vi "Source_Q_wrong.vi"(2 "Ch Names":string[](array[string]), 3 "Values":dbl[](array[numeric]) format="%.2f") -> (0 "Gas Error?":bool)   [LabVIEW 2010]
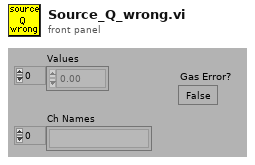
[diagram p1: front panel]
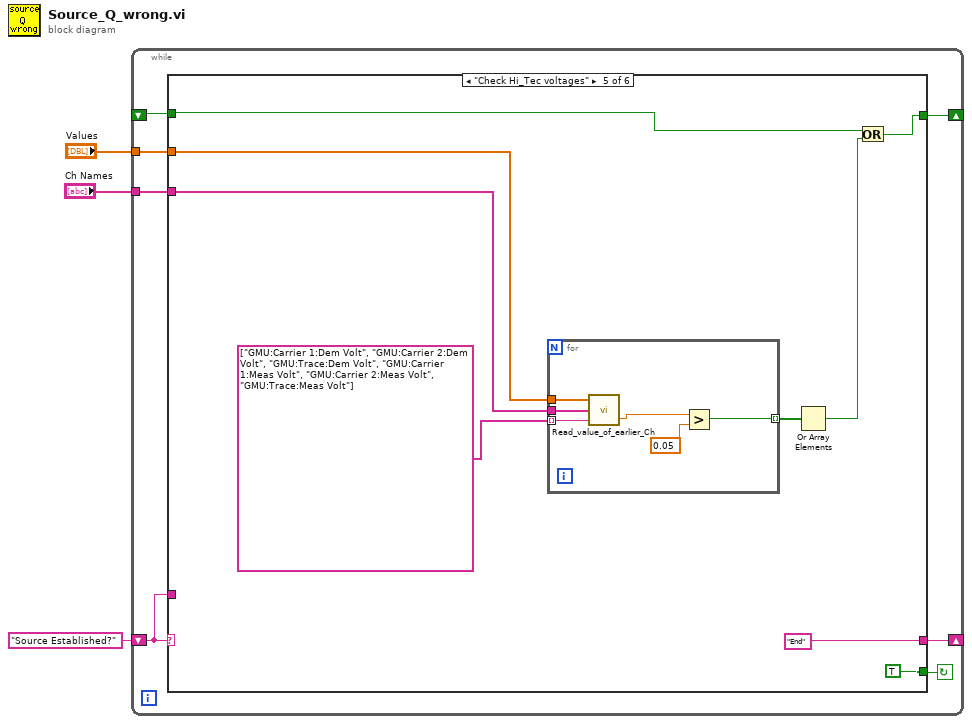
[diagram p0: block diagram]
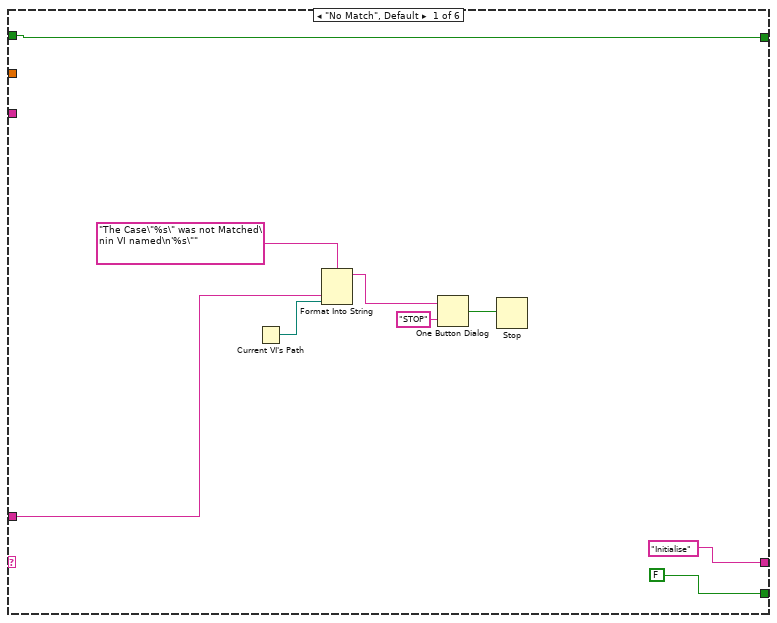
[diagram p2: hidden frame]
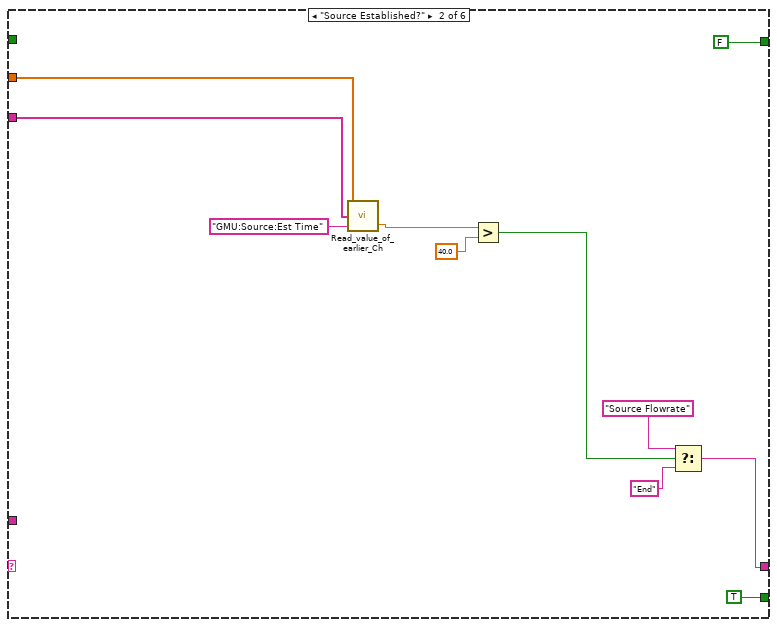
[diagram p3: hidden frame]
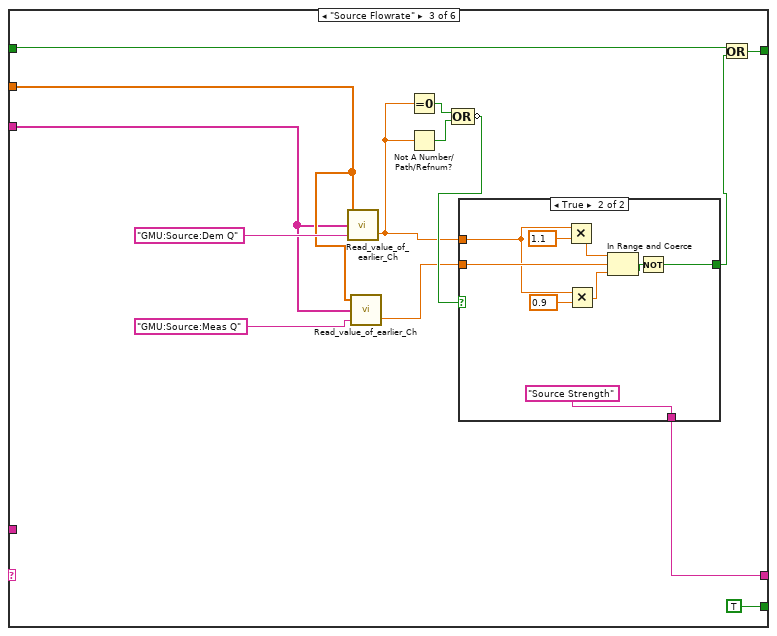
[diagram p4: hidden frame]
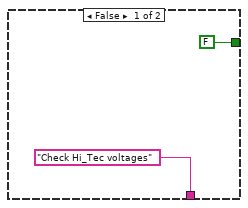
[diagram p5: hidden frame]
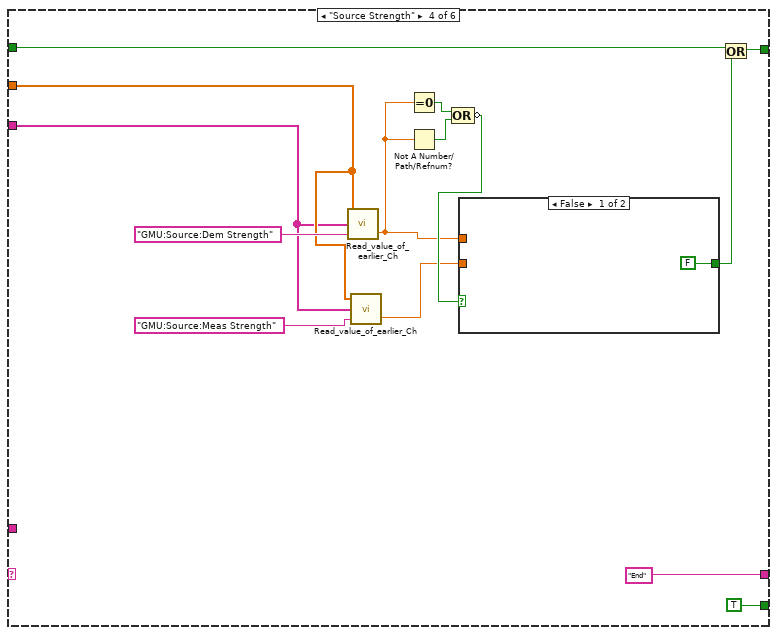
[diagram p6: hidden frame]
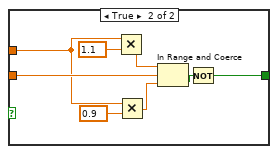
[diagram p7: hidden frame]
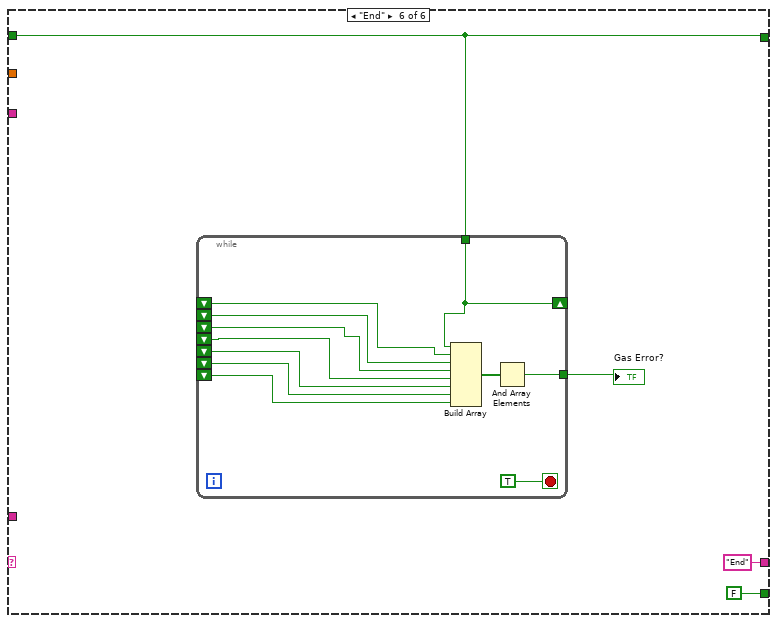
[diagram p8: hidden frame]
diagram:
  n1 = while {
    shift-left: "Source Established?" -> [w8]
    shift-right: [w9] -> _
    tunnel: "Ch Names" -> [w7]
    tunnel: "Values" -> [w6]
    shift-right: [w5] -> _
    shift-left: _ -> [w4]
    stop <- w10 continue-if-true
    n2 = case shown="\"Check Hi_Tec voltages\"" w8 {
      tunnel: [FALSE TRUE TRUE TRUE TRUE FALSE] -> w10
      tunnel: ["Initialise" w21 w31 "End" "End" "End" ("f")] -> w9
      tunnel: w8 -> [w14 _ _ _ _ _]
      tunnel: w7 -> [_ w29 w42 w66 w85 _]
      tunnel: w6 -> [_ w28 w43 w67 w83 _]
      tunnel: [w11 FALSE w34 w56 w79 w95] -> w5
      tunnel: w4 -> [w11 _ w32 w57 w80 w95]
      frame "No Match", Default {
        n3 = Current VI's Path() -> (path=w13:path)
        n4 = Format Into String(format string="The Case\"%s\" was not Matched\nin VI named\n'%s\"" ("Format String"), w14, w13) -> (resulting string=w17:string)  [unwired: 2 in, 1 out]
        n5 = One Button Dialog(message=w17, button name ("OK")="STOP") -> (true=w15:bool)
        n6 = Stop(stop? (T)=w15) -> ()
      }
      frame "Source Established?" {
        n7 = call "Read_value_of_earlier_Ch.vi"("Desired Ch to Read"="GMU:Source:Est Time", "Ch names"=w29, "Present scan array"=w28) -> ("Value"=w26:dbl)  [unwired: 1 in, 1 out]
        n8 = Greater?(x=w26, y=40.0) -> (0:w23:bool)
        n9 = Select(t="Source Flowrate", s=w23, f="End") -> (s? t:f=w21:string)
      }
      frame "Source Flowrate" {
        n10 = call "Read_value_of_earlier_Ch.vi"("Desired Ch to Read"="GMU:Source:Dem Q", "Ch names"=w42, "Present scan array"=w43) -> ("Value"=w37:dbl)  [unwired: 1 in, 1 out]
        n11 = call "Read_value_of_earlier_Ch.vi"("Desired Ch to Read"="GMU:Source:Meas Q", "Ch names"=w42, "Present scan array"=w43) -> ("Value"=w36:dbl)  [unwired: 1 in, 1 out]
        n12 = Equal To 0?(x=w37) -> (x = 0?=w40:bool)
        n13 = Not A Number/Path/Refnum?(number/path/refnum=w37) -> (NaN/Path/Refnum?=w39:bool)
        n14 = Compound Arithmetic op=OR(w40, w39) -> (invert w38:bool)
        n15 = case shown="True" w38 {
          tunnel: w36 -> [_ w51]
          tunnel: w37 -> [_ w50]
          tunnel: [FALSE w48] -> w33
          tunnel: ["Check Hi_Tec voltages" "Source Strength"] -> w31
          frame False {
          }
          frame True {
            n16 = Multiply(x=w50, y=1.1) -> (x*y=w55:dbl)
            n17 = Multiply(x=w50, y=0.9) -> (x*y=w54:dbl)
            n18 = In Range and Coerce(upper limit=w55, x=w51, lower limit=w54) -> (In Range?=w49:bool)  [unwired: 1 out]
            n19 = Not(x=w49) -> (.not. x?=w48:bool)
          }
        }
        n20 = Or(x=w32, y=w33) -> (x .or. y?=w34:bool)
      }
      frame "Source Strength" {
        n21 = call "Read_value_of_earlier_Ch.vi"("Desired Ch to Read"="GMU:Source:Dem Strength", "Ch names"=w66, "Present scan array"=w67) -> ("Value"=w61:dbl)  [unwired: 1 in, 1 out]
        n22 = call "Read_value_of_earlier_Ch.vi"("Desired Ch to Read"="GMU:Source:Meas Strength", "Ch names"=w66, "Present scan array"=w67) -> ("Value"=w60:dbl)  [unwired: 1 in, 1 out]
        n23 = Equal To 0?(x=w61) -> (x = 0?=w64:bool)
        n24 = Not A Number/Path/Refnum?(number/path/refnum=w61) -> (NaN/Path/Refnum?=w63:bool)
        n25 = Compound Arithmetic op=OR(w64, w63) -> (invert w62:bool)
        n26 = case shown="False" w62 {
          tunnel: w60 -> [_ w74]
          tunnel: w61 -> [_ w73]
          tunnel: [FALSE w71] -> w58
          frame False {
          }
          frame True {
            n27 = Multiply(x=w73, y=1.1) -> (x*y=w78:dbl)
            n28 = Multiply(x=w73, y=0.9) -> (x*y=w77:dbl)
            n29 = In Range and Coerce(upper limit=w78, x=w74, lower limit=w77) -> (In Range?=w72:bool)  [unwired: 1 out]
            n30 = Not(x=w72) -> (.not. x?=w71:bool)
          }
        }
        n31 = Or(x=w57, y=w58) -> (x .or. y?=w56:bool)
      }
      frame "Check Hi_Tec voltages" {
        n32 = for {
          tunnel: w83 -> [w93]
          tunnel: w85 -> [w92]
          tunnel: string[] ["GMU:Carrier 1:Dem Volt", "GMU:Carrier 2:Dem Volt", "GMU:Trace:Dem Volt", "GMU:Carrier 1:Meas Volt", "GMU:Carrier 2:Meas Volt", "GMU:Trace:Meas Volt"] ("appended array") -> [w91] mode=indexing
          tunnel: [w88] -> w82 mode=indexing
          n33 = call "Read_value_of_earlier_Ch.vi"("Desired Ch to Read"=w91, "Ch names"=w92, "Present scan array"=w93) -> ("Value"=w89:dbl)  [unwired: 1 in, 1 out]
          n34 = Greater?(x=w89, y=0.05) -> (0:w88:bool)
        }
        n35 = Or Array Elements(Boolean array=w82) -> (logical OR=w81:bool)
        n36 = Or(x=w80, y=w81) -> (x .or. y?=w79:bool)
      }
      frame "End" {
        n37 = while {
          shift-right: [w107] -> _
          shift-left: _ -> [w106]
          shift-left: _ -> [w105]
          shift-left: _ -> [w104]
          shift-left: _ -> [w103]
          shift-left: _ -> [w102]
          shift-left: _ -> [w101]
          shift-left: _ -> [w100]
          tunnel: w95 -> [w107]
          tunnel: [w98] -> w97
          stop <- TRUE stop-if-true
          n38 = Build Array(w107, w106, w105, w104, w103, w102, w101, w100) -> (w99:bool[])
          n39 = And Array Elements(Boolean array=w99) -> (logical AND=w98:bool)
        }
        "Gas Error?" <- w97
      }
    }
  }
